vi "AcquireData.vi"(6 "ScanEnable":bool, 7 "DataIn":sgl[](array[numeric]), 8 "error in":errorcluster, 9 "linesPerUpdate":u16, 10 "Pixels/Line":u32, 11 "FPGA VI Reference In":T1) -> (0 "error out":errorcluster, 1 "BlockUpdate?":bool, 2 "Elements Remaining":u32, 3 "FPGA VI Reference Out":T1, 5 "DataOut":sgl[](array[numeric]))   [LabVIEW 2016]
doc: "Acquires the data from the FPGA and packages it in the FGV Data."
uses:
  controls/FPGAVIreferenceTypeDef.ctl
  <vilib>/rvi/errors/niLvFpgaAdjustHostInterfaceError.vi
  <vilib>/Utility/error.llb/Error Cluster From Error Code.vi
  <vilib>/rvi/interface/nirviMethod/nirviMethod.xnode
  FPGA Bitfiles/qnmController797_usbRIO_controllerFPGAmu.lvbitx
  <vilib>/rvi/errors/niLvFpgaMergeErrorWithErrorCode.vi
  <vilib>/FPGAPlugInAG/USB-7856R OEM/niLvFpga_ReadFifo_USB-7856R OEM.vi
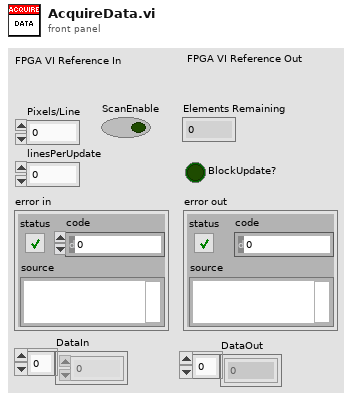
[diagram p1: front panel]
types:
  T1 = typedef "FPGAVIreferenceTypeDef.ctl" = refnum<k20>
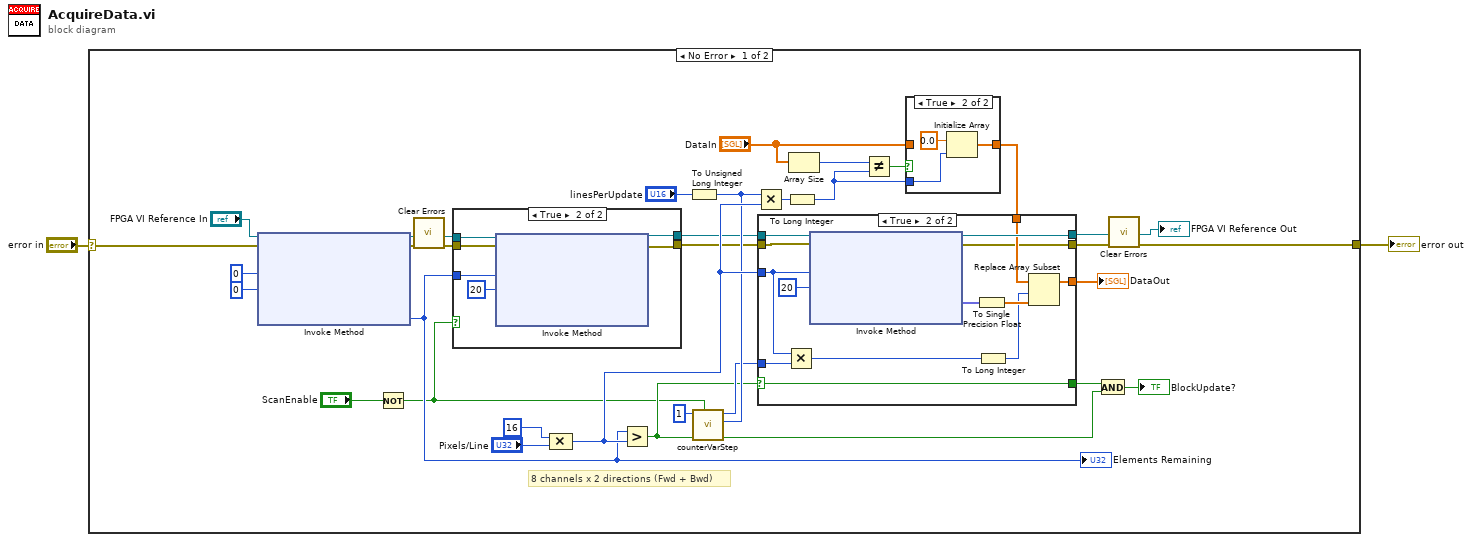
[diagram p0: block diagram]
diagram:
  n1 = case shown="No Error" "error in" {
    selector: "error in" -> [w3 w66]
    tunnel: [w4 w66] -> w2
    frame No Error {
      # "8 channels x 2 directions (Fwd + Bwd)"
      n2 = xnode "Invoke Method"("FPGA VI Reference In"="FPGA VI Reference In", "error in"=w3, "Number of Elements"=u32 0, "Timeout (ms)"=0) -> ("FPGA VI Reference Out"=w14:T1, "error out"=w8:errorcluster, "Elements Remaining"=w21:u32)  [unwired: 1 out]
      "Elements Remaining" <- w21
      n3 = Not(x="ScanEnable") -> (.not. x?=w20:bool)
      n4 = call <vilib>:"Clear Errors.vi"("error in (no error)"=w8) -> ("error out"=w5:errorcluster)  [unwired: 5 in, 1 out]
      n5 = case shown="True" w20 {
        tunnel: w14 -> [w59 w62]
        tunnel: w21 -> [_ w64]
        tunnel: [w59 w65] -> w29
        tunnel: w5 -> [w58 w61]
        tunnel: [w58 w60] -> w7
        frame False {
        }
        frame True {
          n6 = xnode "Invoke Method"("FPGA VI Reference In"=w62, "error in"=w61, "Number of Elements"=w64, "Timeout (ms)"=20) -> ("FPGA VI Reference Out"=w65:T1, "error out"=w60:errorcluster)  [unwired: 2 out]
        }
      }
      n7 = Compound Arithmetic op=MULTIPLY(u32 16 ("x"), "Pixels/Line") -> (w35:u32)
      n8 = Greater?(x=w21, y=w35) -> (0:w25:bool)
      n9 = To Unsigned Long Integer(number="linesPerUpdate") -> (unsigned 32bit integer=w30:u32)
      n10 = call "counterVarStep.vi"("stepSize"=u32 1, "countMax"=w30, "doStep"=w25, "reset"=w20) -> ("index"=w28:u32, "maxReached"=w32:bool)  [unwired: 4 in, 1 out]
      n11 = Multiply(x=w30, y=w35) -> (x*y=w26:u32)
      n12 = To Long Integer(number=w26) -> (32bit integer=w12:i32)
      n13 = Array Size(array="DataIn") -> (size(s)=w13:i32)
      n14 = Not Equal?(x=w13, y=w12) -> (x != y?=w18:bool)
      n15 = case shown="True" w18 {
        tunnel: w12 -> [_ w39]
        tunnel: [w36 w37] -> w27
        tunnel: "DataIn" -> [w36 _]
        frame False {
        }
        frame True {
          n16 = Initialize Array(sgl 0.0 ("element"), w39) -> (w37:sgl[])
        }
      }
      n17 = case shown="True" w25 {
        selector: w25 -> [w42 w52]
        tunnel: w29 -> [w41 w57]
        tunnel: w35 -> [_ w50]
        tunnel: [w41 w56] -> w22
        tunnel: [w43 w55] -> w19
        tunnel: w27 -> [w43 w54]
        tunnel: w28 -> [_ w51]
        tunnel: [w42 w52] -> w31
        tunnel: w7 -> [w40 w45]
        tunnel: [w40 w44] -> w6
        frame False {
        }
        frame True {
          n18 = Multiply(x=w50, y=w51) -> (x*y=w53:u32)
          n19 = xnode "Invoke Method"("FPGA VI Reference In"=w57, "error in"=w45, "Number of Elements"=w50, "Timeout (ms)"=20) -> ("FPGA VI Reference Out"=w56:T1, "error out"=w44:errorcluster, "Data"=w47:fxp<+/-,18,1>[])  [unwired: 1 out]
          n20 = To Single Precision Float(number=w47) -> (single precision float=w48:sgl[])
          n21 = To Long Integer(number=w53) -> (32bit integer=w46:i32)
          n22 = Replace Array Subset(array=w54, new element=w48, index=w46) -> (w55:sgl[])
        }
      }
      "FPGA VI Reference Out" <- w22
      "DataOut" <- w19
      n23 = And(x=w31, y=w32) -> (x .and. y?=→"BlockUpdate?":bool)
      n24 = call <vilib>:"Clear Errors.vi"("error in (no error)"=w6) -> ("error out"=w4:errorcluster)  [unwired: 5 in, 1 out]
    }
    frame Error {
    }
  }
  "error out" <- w2
